vi "scan2d_generate_UI_events.vi"(8 "error in (no error)":errorcluster, 11 "scan_panel in":refnum<class "scan_2d.lvclass">) -> (0 "error out":errorcluster, 2 "update_status":refnum<event-registration>, 3 "scan_panel out":refnum<class "scan_2d.lvclass">)   [LabVIEW 2015, in "scan_2d.lvclass"]
uses:
  scan_2d.lvclass
  Scan/scan_ui_event_references.ctl
  Scan/scan_ui_events.ctl
  scan_2d.lvclass/scan_2d.ctl
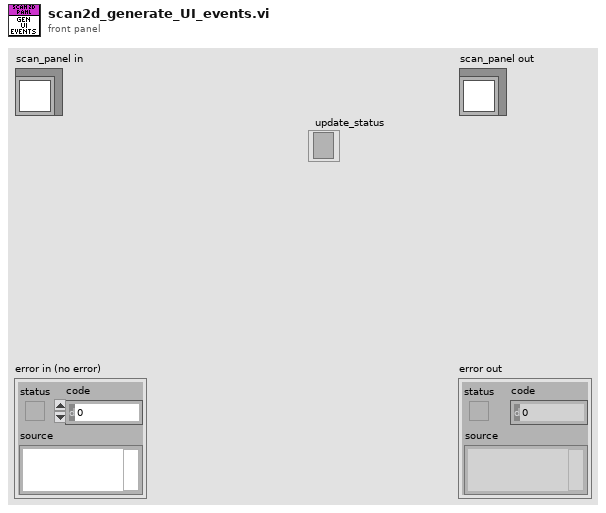
[diagram p1: front panel]
types:
  T1 = typedef "scan_ui_events.ctl" = cluster{"update_scan_status":refnum<user-event>}
  T2 = typedef "scan_ui_event_references.ctl" = cluster{"update_status_string_":refnum<event-registration>}
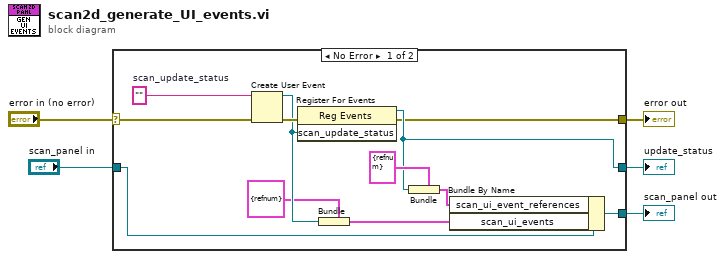
[diagram p0: block diagram]
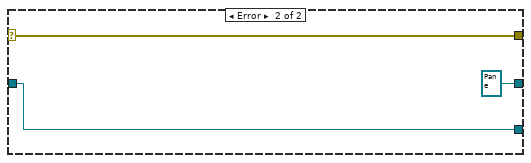
[diagram p2: hidden frame]
diagram:
  n1 = case shown="No Error" "error in (no error)" {
    selector: "error in (no error)" -> [w17 w20]
    tunnel: [w6 w20] -> w4
    tunnel: [w10 w19] -> w2
    tunnel: "scan_panel in" -> [w12 w19]
    tunnel: [w13 refnum<event-registration> refnum ("Event Registration Refnum")] -> w1
    frame No Error {
      w16 = ""  # scan_update_status
      n2 = Create User Event(user event datatype=w16, error in=w17) -> (user event=w9:refnum<user-event>, error out=w15:errorcluster)
      n3 = register-events(error in=w15, w9) -> (reference out=w13:refnum<event-registration>, error out=w6:errorcluster)  [unwired: 1 in]
      n4 = Bundle(cluster=T1 {"update_scan_status"=refnum} ("output cluster"), "update_scan_status"=w9) -> (w7:T1)
      n5 = Bundle(cluster=T2 {"update_status_string_"=refnum} ("scan_ui_event_references"), "update_status_string_"=w13) -> (w11:T2)
      n6 = Bundle By Name(cluster=w12, "scan_ui_event_references"=w11, "scan_ui_events"=w7) -> (w10:refnum<class "scan_2d.lvclass">)
    }
    frame Error {
    }
  }
  "error out" <- w4
  "scan_panel out" <- w2
  "update_status" <- w1
